vi "Imprimer les n° d'une cmde.vi"(2 "error in (no error)":errorcluster caption="entrée d'erreur (pas d'erreur)", 3 "n° commande":string="6340/07-02.01.01") -> (0 "error IO":errorcluster)   [LabVIEW 2020]
doc: "Enregistre les paramètres d'emballage (DATA3) dans la base de donnée"
uses:
  Modules/FS/60_FS_Controles/60_FS_SetGet.ctl
  <vilib>/Utility/NIReport.llb/NI_ReportGenerationCore.lvlib
  <vilib>/Utility/NIReport.llb/NI_report.lvclass
panel:
  out "Indice Rev. Client":string
  out "N° article Client":string
  in  "CreerFichierSpec":bool
  out "Glissière 2":u8(slide)=100 caption="Identification terminé." scale=0.0..100.0
  in  "supprimer la commande":bool
  out "Quantité :":string
  in  "quitter":bool
  in  "Fichier généré":string
  in  "IMPRIMER":bool
  in  "Bouton OK":bool
  # "Saisir le n° de la commande à imprimer"
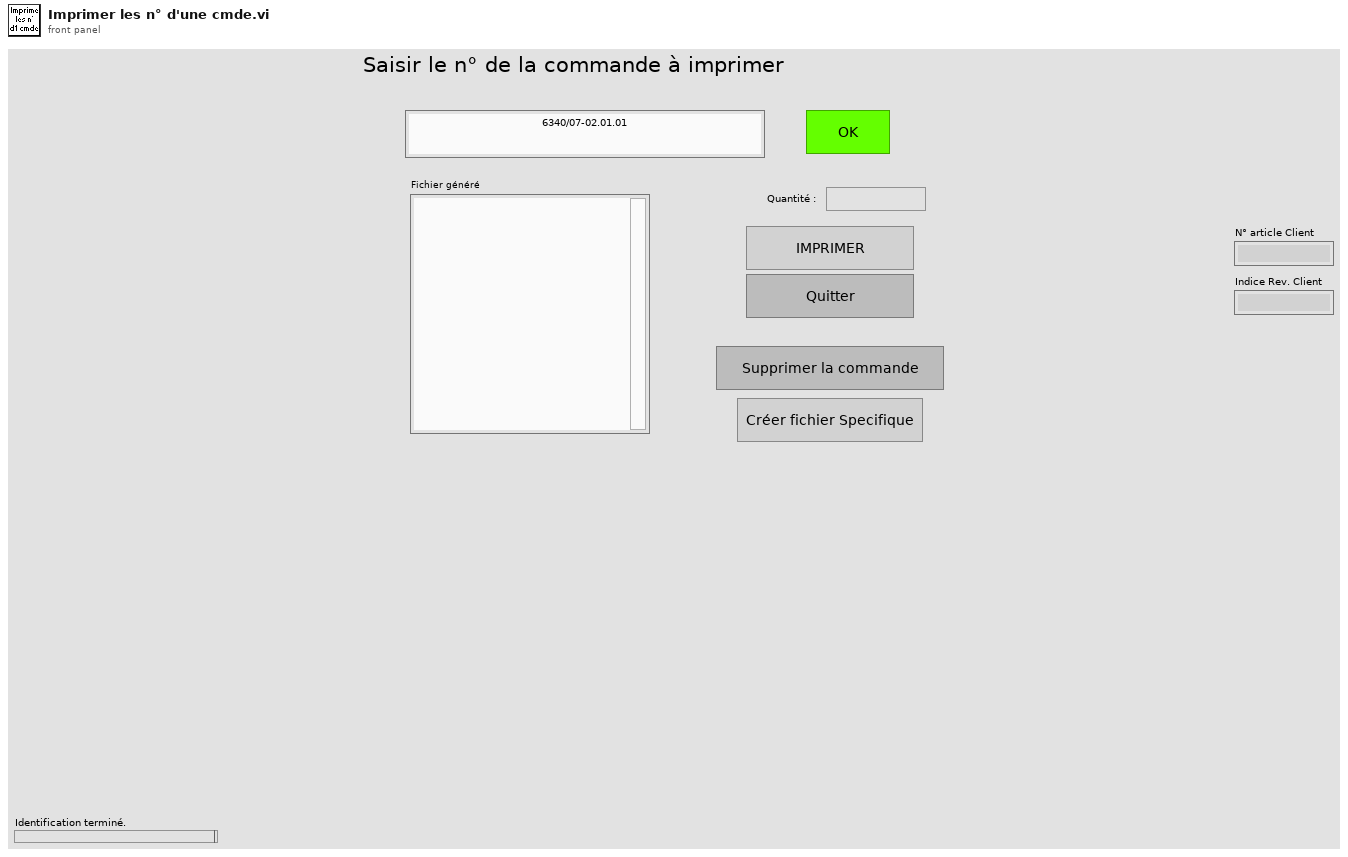
[diagram p1: front panel]
types:
  T1 = enum8{"Enabled", "Disabled", "Disabled and Grayed Out"}
  T2 = typedef "60_FS_SetGet.ctl" = enum16{"set", "get"}
  T3 = typedef "60_FS_CLT_Chemins.ctl" = cluster{"Racine_local":path, "Racine_reseau":path, "Racine_Support_Application":path, "Fichier_Journalisation":path, "Connexion_BDD_VSX":path, "Connexion_BDD_PLZ":path}
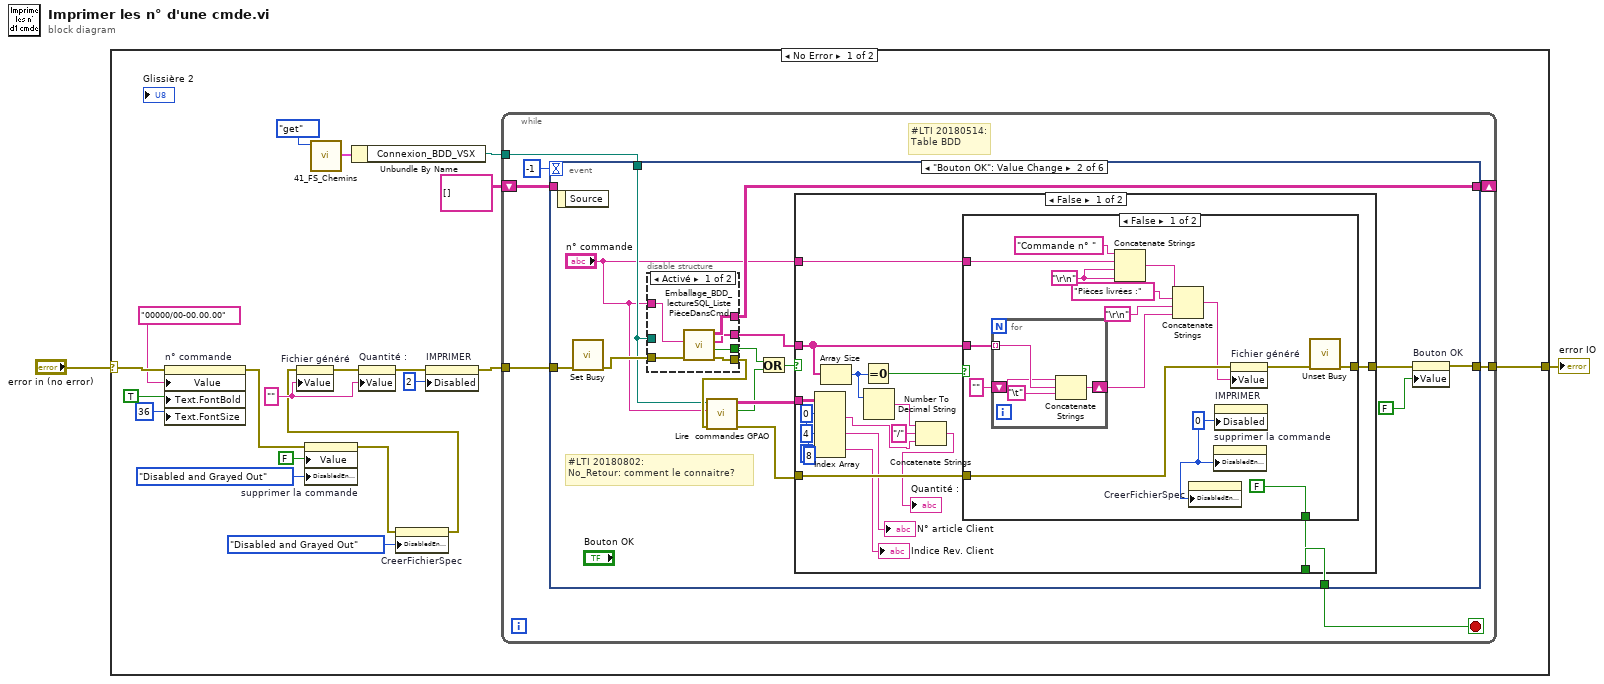
[diagram p0: block diagram]
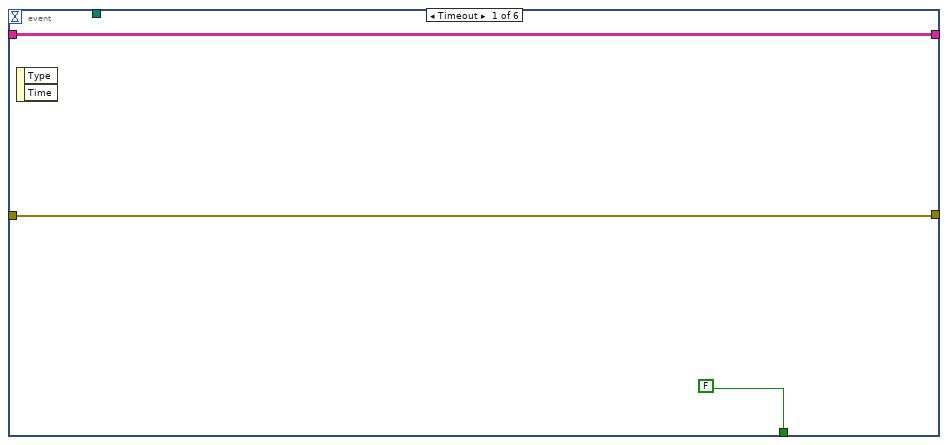
[diagram p2: hidden frame]
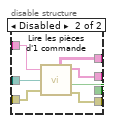
[diagram p3: hidden frame]
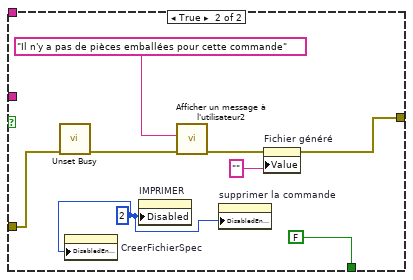
[diagram p4: hidden frame]
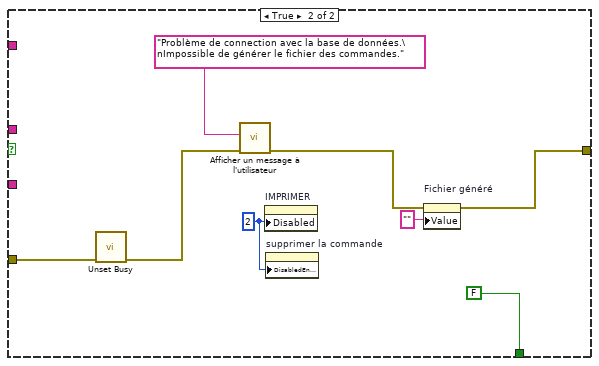
[diagram p5: hidden frame]
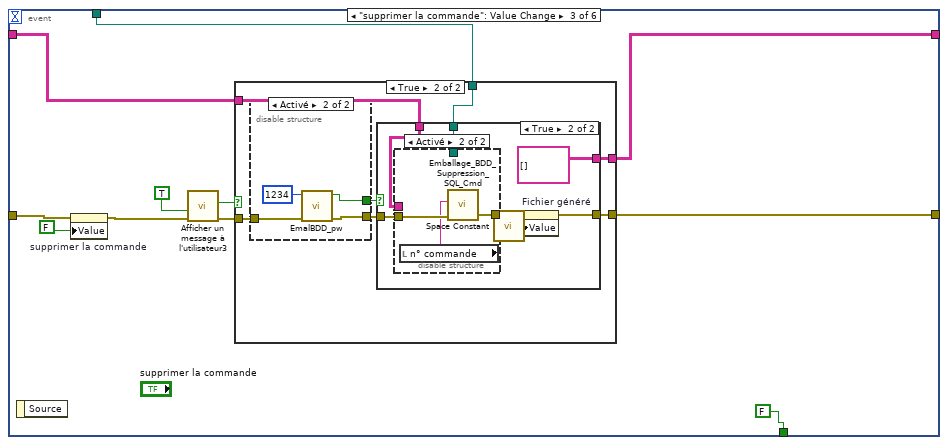
[diagram p6: hidden frame]
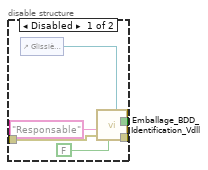
[diagram p8: hidden frame]
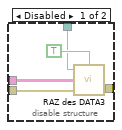
[diagram p10: hidden frame]
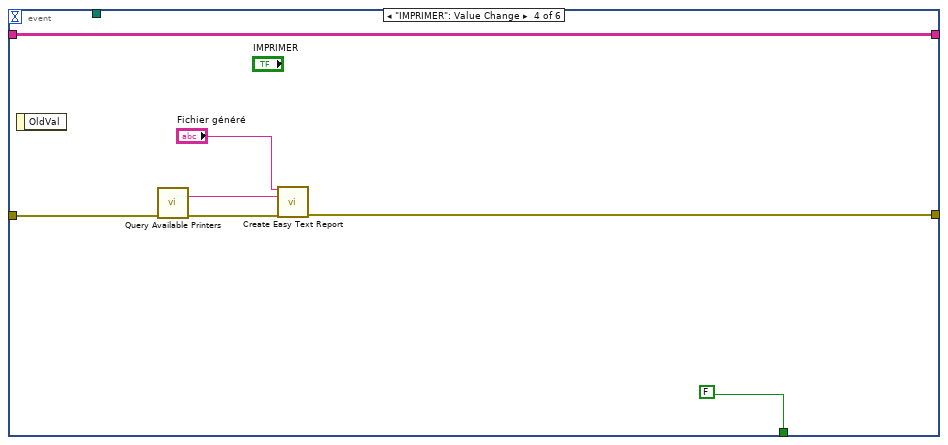
[diagram p11: hidden frame]
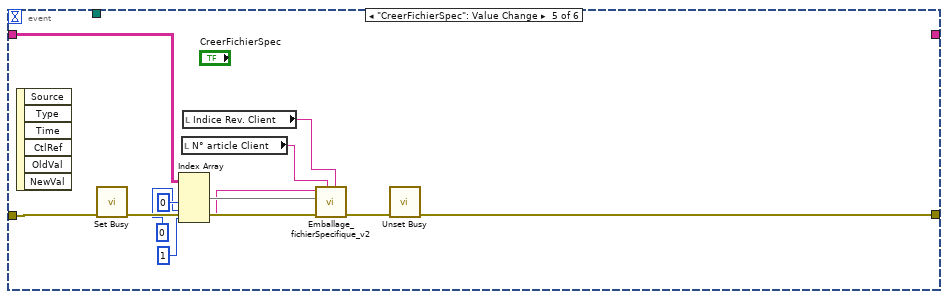
[diagram p12: hidden frame]
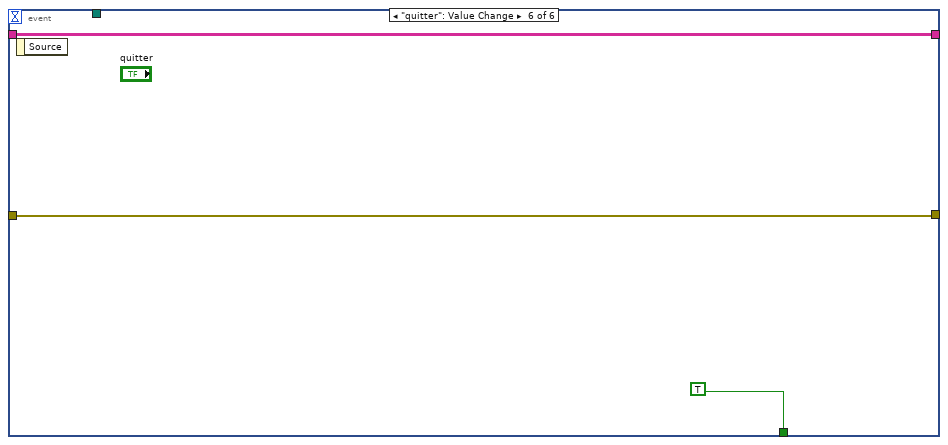
[diagram p13: hidden frame]
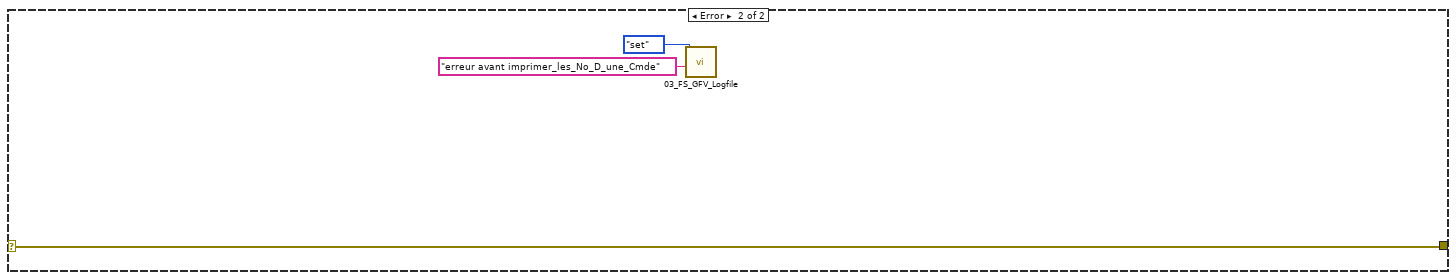
[diagram p14: hidden frame]
diagram:
  n1 = case shown="No Error" "error in (no error)" {
    selector: "error in (no error)" -> [w22 w186]
    tunnel: [w18 w186] -> w1
    frame No Error {
      w13 = "" ("n° commande")
      n2 = property on="n° commande" class="Str"(error in=w22, "Value"="00000/00-00.00.00" ("n° commande"), "Text.FontBold"=TRUE ("Texte.Police : gras"), "Text.FontSize"=u32 36 ("Texte.Police : taille")) -> (error out=w12:errorcluster)  [unwired: 1 in, 1 out]
      n3 = property on="supprimer la commande" class="Bool (strict)"(error in=w12, "Value"=FALSE ("supprimer la commande"), "DisabledEnum"=T1."Disabled and Grayed Out" ("Désactivé")) -> (error out=w4:errorcluster)  [unwired: 1 in, 1 out]
      n4 = call "41_FS_Chemins.vi"("SetGet"=60_FS_SetGet."get") -> ("CLT_Chemins_out"=w9:T3)  [unwired: 9 in, 1 out]
      n5 = Unbundle By Name(w9) -> ("Connexion_BDD_VSX"=w8:path)
      n6 = property on="CreerFichierSpec" class="Bool"(error in=w4, "DisabledEnum"=T1."Disabled and Grayed Out" ("Désactivé")) -> (error out=w3:errorcluster)  [unwired: 1 in, 1 out]
      n7 = property on="Fichier généré" class="Str"(error in=w3, "Value"=w13) -> (error out=w15:errorcluster)  [unwired: 1 in, 1 out]
      n8 = property on="Quantité :" class="Str"(error in=w15, "Value"=w13) -> (error out=w14:errorcluster)  [unwired: 1 in, 1 out]
      n9 = property on="IMPRIMER" class="Bool"(error in=w14, "Disabled"=u8 2 ("Désactivé")) -> (error out=w19:errorcluster)  [unwired: 1 in, 1 out]
      n10 = while {
        tunnel: w19 -> [w29]
        tunnel: [w27] -> w18
        shift-right: [w26] -> _
        shift-left: string[][] [] ("Tableau") -> [w25]
        tunnel: w8 -> [w23]
        stop <- w28 stop-if-true
        # "#LTI 20180514:\nTable BDD"
        n11 = event shown="[1] \"Bouton OK\": Value Change" {
          selector: _ -> [_ _ _ _ _ _]
          dyn-events: _ -> [_ _ _ _ _ _]
          timeout: -1 -> [_ _ _ _ _ _]
          tunnel: w29 -> [w31 w47 w125 w167 w180 w182]
          tunnel: [w31 w38 w119 w164 w174 w182] -> w27
          tunnel: [FALSE w48 FALSE FALSE _ TRUE] -> w28
          tunnel: w23 -> [_ w34 w115 _ _ _]
          tunnel: [w30 w35 w117 w163 _ w181] -> w26
          tunnel: w25 -> [w30 _ w116 w163 w178 w181]
          event Timeout {
            n12 = event-data() -> ()  [unwired: 1 in, 2 out]
          }
          event "Bouton OK": Value Change {
            # "#LTI 20180802:\nNo_Retour: comment le connaitre?"
            n13 = event-data() -> ()  [unwired: 1 in, 1 out]
            n14 = call <vilib>:"Set Busy.vi"("error in (no error)"=w47) -> ("error out"=w46:errorcluster)  [unwired: 9 in, 1 out]
            n15 = disable-structure shown="Activé" {
              disable-tunnel: w46 -> [w54 w61]
              disable-tunnel: [w53 w60] -> w45
              disable-tunnel: "n° commande" -> [w52 w58]
              disable-tunnel: [w49 w55] -> w40
              disable-tunnel: [w50 w56] -> w36
              disable-tunnel: [w51 w59] -> w35
              disable-tunnel: w34 -> [_ w57]
              frame Enabled {
                n16 = call "Emballage_BDD_lectureSQL_Liste PièceDansCmd.vi"("Error in"=w54, "NO_CDEVAL"=w52) -> ("Error out"=w53:errorcluster, "Erreur de  comunication"=w49:bool, "Liste n° pièces de la cmde"=w50:string[], "Donnees"=w51:string[][])  [unwired: 5 in, 1 out]
              }
              frame Disabled {
                n17 = call "Lire les pièces d'1 commande.vi"("n° commande"=w58, "connection information"=w57, "error in (no error)"=w61) -> ("Liste n° pièces de la cmde"=w56:string[], "Erreur de\n comunication"=w55:bool, "error out"=w60:errorcluster, "Tableau"=w59:string[][])  [unwired: 1 out]
              }
            }
            n18 = call "Lire  commandes GPAO.vi"("error in"=w45, "Numéro commande"="n° commande", "connection information"=w34) -> ("error out"=w44:errorcluster, "Erreur de\n comunication"=w41:bool, "Tab cmde GPAO"=w43:string[][])  [unwired: 4 in, 2 out]
            n19 = Or(x=w40, y=w41) -> (x .or. y?=w42:bool)
            n20 = case shown="False" w42 {
              tunnel: w36 -> [w75 _]
              tunnel: w44 -> [w77 w109]
              tunnel: [w78 w112] -> w39
              tunnel: "n° commande" -> [w79 _]
              tunnel: [w76 FALSE] -> w48
              tunnel: w43 -> [w73 _]
              frame False {
                w65 = 0 ("indice désactivé (ligne)")
                n21 = Index Array(array=w73, index (row) #1=w65, index (col) #1=4 ("indice désactivé (col)"), index (row) #2=w65, index (col) #2=8 ("indice désactivé (col)"), index (row) #3=w65, index (col) #3=9 ("indice désactivé (col)")) -> (element #1=w69:string, element #2=→"N° article Client":string, element #3=→"Indice Rev. Client":string)
                n22 = Array Size(array=w75) -> (size(s)=w71:i32)
                n23 = Equal To 0?(x=w71) -> (x = 0?=w74:bool)
                n24 = Number To Decimal String(number=w71) -> (decimal integer string=w70:string)  [unwired: 1 in]
                n25 = Concatenate Strings(w70, "/" ("chaîne"), w69) -> (→"Quantité :":string)
                n26 = case shown="False" w74 {
                  tunnel: w79 -> [w93 _]
                  tunnel: [w81 w101] -> w78
                  tunnel: w75 -> [w90 _]
                  tunnel: w77 -> [w88 w104]
                  tunnel: [FALSE FALSE] -> w76
                  frame False {
                    w80 = u8 0 ("Désactivé")
                    w92 = "\r\n"
                    n27 = for {
                      tunnel: w90 -> [w97] mode=indexing
                      shift-right: [w96] -> w85
                      shift-left: "" -> [w95]
                      n28 = Concatenate Strings(w95, w97, "\t") -> (w96:string)
                    }
                    n29 = Concatenate Strings("Commande n° " ("n° commande"), w93, w92, w92) -> (w87:string)
                    n30 = Concatenate Strings(w87, "Pièces livrées :" ("n° commande"), "\r\n", w85) -> (w86:string)
                    n31 = property on="CreerFichierSpec" class="Bool"("DisabledEnum"=w80) -> ()  [unwired: 2 in, 2 out]
                    n32 = property on="supprimer la commande" class="Bool (strict)"("DisabledEnum"=w80) -> ()  [unwired: 2 in, 2 out]
                    n33 = property on="IMPRIMER" class="Bool"("Disabled"=w80) -> ()  [unwired: 2 in, 2 out]
                    n34 = property on="Fichier généré" class="Str"(error in=w88, "Value"=w86) -> (error out=w82:errorcluster)  [unwired: 1 in, 1 out]
                    n35 = call <vilib>:"Unset Busy.vi"("error in (no error)"=w82) -> ("error out"=w81:errorcluster)  [unwired: 10 in]
                  }
                  frame True {
                    w99 = u8 2 ("Désactivé")
                    n36 = call <vilib>:"Unset Busy.vi"("error in (no error)"=w104) -> ("error out"=w103:errorcluster)  [unwired: 10 in]
                    n37 = property on="CreerFichierSpec" class="Bool"("DisabledEnum"=w99) -> ()  [unwired: 2 in, 2 out]
                    n38 = property on="IMPRIMER" class="Bool"("Disabled"=w99) -> ()  [unwired: 2 in, 2 out]
                    n39 = call "Afficher un message à l'utilisateur2"("error in (no error)"=w103, "Message"="Il n'y a pas de pièces emballées pour cette commande") -> ("error out"=w102:errorcluster)  [unwired: 8 in, 1 out]
                    n40 = property on="supprimer la commande" class="Bool (strict)"("DisabledEnum"=w99) -> ()  [unwired: 2 in, 2 out]
                    n41 = property on="Fichier généré" class="Str"(error in=w102, "Value"="" ("Fichier généré")) -> (error out=w101:errorcluster)  [unwired: 1 in, 1 out]
                  }
                }
              }
              frame True {
                w107 = u8 2 ("Désactivé")
                n42 = call <vilib>:"Unset Busy.vi"("error in (no error)"=w109) -> ("error out"=w108:errorcluster)  [unwired: 10 in]
                n43 = call "Afficher un message à l'utilisateur"("error in (no error)"=w108, "Message"="Problème de connection avec la base de données.\nImpossible de générer le fichier des commandes.") -> ("error out"=w113:errorcluster)  [unwired: 8 in, 1 out]
                n44 = property on="IMPRIMER" class="Bool"("Disabled"=w107) -> ()  [unwired: 2 in, 2 out]
                n45 = property on="supprimer la commande" class="Bool (strict)"("DisabledEnum"=w107) -> ()  [unwired: 2 in, 2 out]
                n46 = property on="Fichier généré" class="Str"(error in=w113, "Value"="" ("Pièces emballées sous cette commande")) -> (error out=w112:errorcluster)  [unwired: 1 in, 1 out]
              }
            }
            n47 = property on="Bouton OK" class="Bool (strict)"(error in=w39, "Value"=FALSE ("Bouton OK")) -> (error out=w38:errorcluster)  [unwired: 1 in, 1 out]
          }
          event "supprimer la commande": Value Change {
            n48 = event-data() -> ()  [unwired: 1 in, 1 out]
            n49 = property on="supprimer la commande" class="Bool (strict)"(error in=w125, "Value"=FALSE ("supprimer la commande")) -> (error out=w123:errorcluster)  [unwired: 1 in, 1 out]
            n50 = call "Afficher un message à l'utilisateur3"("error in (no error)"=w123, "Enable"=TRUE) -> ("error out"=w122:errorcluster, "Effacer"=w120:bool)  [unwired: 8 in]
            n51 = case shown="True" w120 {
              tunnel: w122 -> [w127 w133]
              tunnel: [w127 w132] -> w119
              tunnel: [w126 w130] -> w117
              tunnel: w116 -> [w126 w129]
              tunnel: w115 -> [_ w128]
              frame False {
              }
              frame True {
                n52 = disable-structure shown="Activé" {
                  disable-tunnel: [w137 w142] -> w134
                  disable-tunnel: w133 -> [w136 w143]
                  disable-tunnel: [w135 w141] -> w131
                  frame Disabled {
                    n53 = control-ref of="Glissière 2"() -> (w140:refnum<vi>)
                    n54 = call "Emballage_BDD_Identification_Vdll.vi"("Glissière"=w140, "lecture seul possible ?"=FALSE, "error in"=w136, "Posage choisi"="Responsable" ("Posage choissi")) -> ("error Out"=w137:errorcluster, "OK"=w135:bool)  [unwired: 3 in, 3 out]
                  }
                  frame Enabled {
                    n55 = call "EmalBDD_pw.vi"("Error in"=w143, "PWattendu"=u32 1234) -> ("Error Out"=w142:errorcluster, "pwOK?"=w141:bool)  [unwired: 8 in]
                  }
                }
                n56 = case shown="True" w131 {
                  tunnel: w134 -> [w146 w153]
                  tunnel: [w146 w149] -> w132
                  tunnel: [w145 string[][] [] ("Tableau")] -> w130
                  tunnel: w129 -> [w145 w152]
                  tunnel: w128 -> [_ w147]
                  frame False {
                  }
                  frame True {
                    n57 = disable-structure shown="Activé" {
                      disable-tunnel: w153 -> [w157 w161]
                      disable-tunnel: w152 -> [w156 _]
                      disable-tunnel: [w155 w160] -> w150
                      disable-tunnel: w147 -> [w154 _]
                      frame Disabled {
                        n58 = call "RAZ des DATA3.vi"("Activer ?"=TRUE, "error in (no error)"=w157, "Tab n° valves à effacer"=w156, "connection information"=w154) -> ("error out 2"=w155:errorcluster)  [unwired: 1 out]
                      }
                      frame Enabled {
                        n59 = local read "n° commande"() -> (w159:string)
                        n60 = call "Emballage_BDD_Suppression_SQL_Cmd.vi"("error in (no error)"=w161, "NO_CDEVAL"=w159) -> ("error out"=w160:errorcluster)  [unwired: 9 in]
                      }
                    }
                    n61 = call <vilib>:"Space Constant.vi"() -> ("String"=w148:string)
                    n62 = property on="Fichier généré" class="Str"(error in=w150, "Value"=w148) -> (error out=w149:errorcluster)  [unwired: 1 in, 1 out]
                  }
                }
              }
            }
          }
          event "IMPRIMER": Value Change {
            n63 = event-data() -> ()  [unwired: 1 in, 1 out]
            n64 = call <vilib>:"Query Available Printers.vi"("error in (no error)"=w167) -> ("error out"=w165:errorcluster, "default printer"=w166:string)  [unwired: 8 in, 1 out]
            n65 = call <vilib>:"Create Easy Text Report.vi"("text to be printed"="Fichier généré", "printer name (default) or file path (dialog)"=w166, "error in (no error)"=w165) -> ("error out"=w164:errorcluster)  [unwired: 12 in]
          }
          event "CreerFichierSpec": Value Change {
            n66 = event-data() -> ()  [unwired: 1 in, 6 out]
            n67 = call <vilib>:"Set Busy.vi"("error in (no error)"=w180) -> ("error out"=w175:errorcluster)  [unwired: 9 in, 1 out]
            n68 = Index Array(array=w178, index (col) #1=0 ("indice désactivé (col)"), index (row) #2=0 ("indice désactivé (ligne)"), index (col) #2=1 ("indice (col)")) -> (element #1=w176:string[], element #2=w171:string)  [unwired: 1 in]
            n69 = local read "N° article Client"() -> (w170:string)
            n70 = local read "Indice Rev. Client"() -> (w169:string)
            n71 = call "Emballage_fichierSpecifique_v2.vi"("Indice Rev. Client"=w169, "N° article client"=w170, "error in (no error)"=w175, "Tableau n° valves"=w176, "Datetime"=w171) -> ("error out"=w179:errorcluster)  [unwired: 6 in]
            n72 = call <vilib>:"Unset Busy.vi"("error in (no error)"=w179) -> ("error out"=w174:errorcluster)  [unwired: 10 in]
          }
          event "quitter": Value Change {
            n73 = event-data() -> ()  [unwired: 1 in, 1 out]
          }
        }
      }
    }
    frame Error {
      n74 = call "03_FS_GFV_Logfile.vi"("Chaîne"="erreur avant imprimer_les_No_D_une_Cmde", "States"=60_FS_SetGet."set") -> ()  [unwired: 8 in, 2 out]
    }
  }
  "error IO" <- w1
